vi "roi_selection multi.vi"(7 "Peak selected":i32, 8 "List Parameter Fit In":dbl[][](array[numeric]), 9 "List ROI In":dbl[][](array[numeric]), 10 "List Peaks":string[][](table), 11 "Spectrum In":cluster{"Locations":dbl[], "Amplitudes":dbl[]}) -> (2 "List Parameter Fit Out":dbl[][](array[numeric]), 3 "List ROI Out":dbl[][](array[numeric]))   [LabVIEW 2020]
uses:
  <vilib>/Analysis/NI_AALPro.lvlib
  <vilib>/Analysis/6fits.llb/Curve Fitting Criteria.ctl
panel:
  out "Parameters Fit":T1
  out "standard deviation":dbl
  out "FWHM":dbl
  out "amplitude":dbl
  out "XY Graph 2":cluster{dbl[], "Best Gaussian Fit":dbl[]}[](graph)
  in  "Elements":string[][](table)
  out "XY Graph":cluster{"Channels":dbl[], "Intensity":dbl[]}(graph)
  out "Spectrum":cluster{"Locations":dbl[], "Amplitudes":dbl[]}(graph)
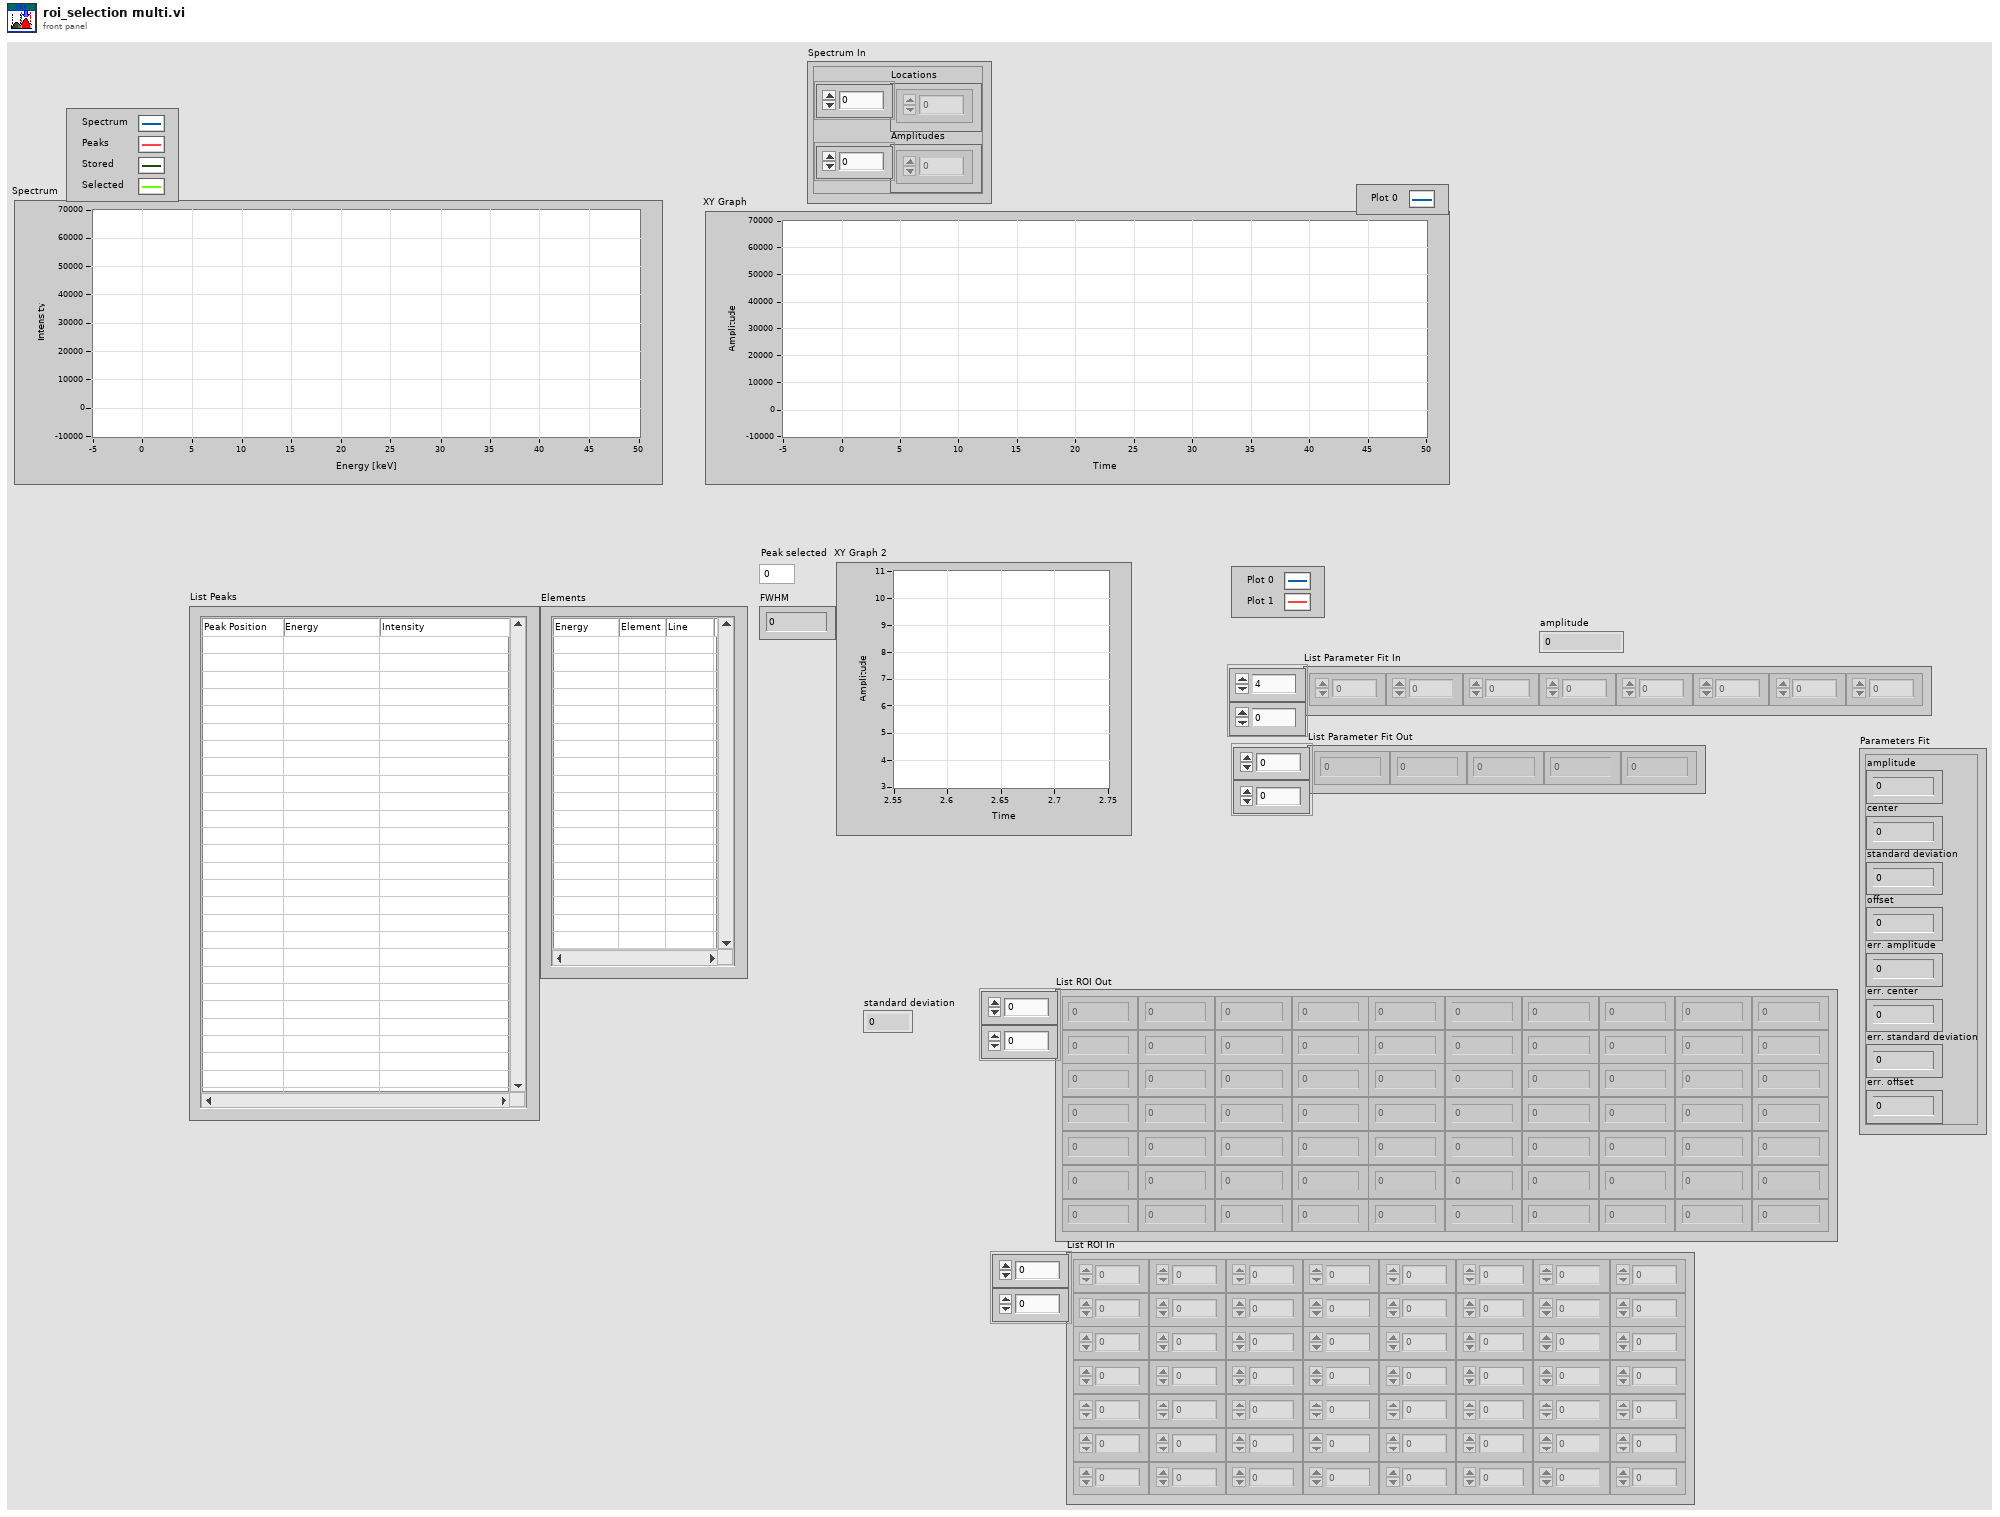
[diagram p1: front panel]
types:
  T1 = cluster{"amplitude":dbl, "center":dbl, "standard deviation":dbl, "offset":dbl, "err. amplitude":dbl, "err. center":dbl, "err. standard deviation":dbl, "err. offset":dbl}
  T2 = cluster{"initial amplitude":dbl, "initial center":dbl, "initial standard deviation":dbl, "offset":dbl}
  T3 = typedef "NI_AALPro.lvlib/Curve Fitting Criteria.ctl" = u16
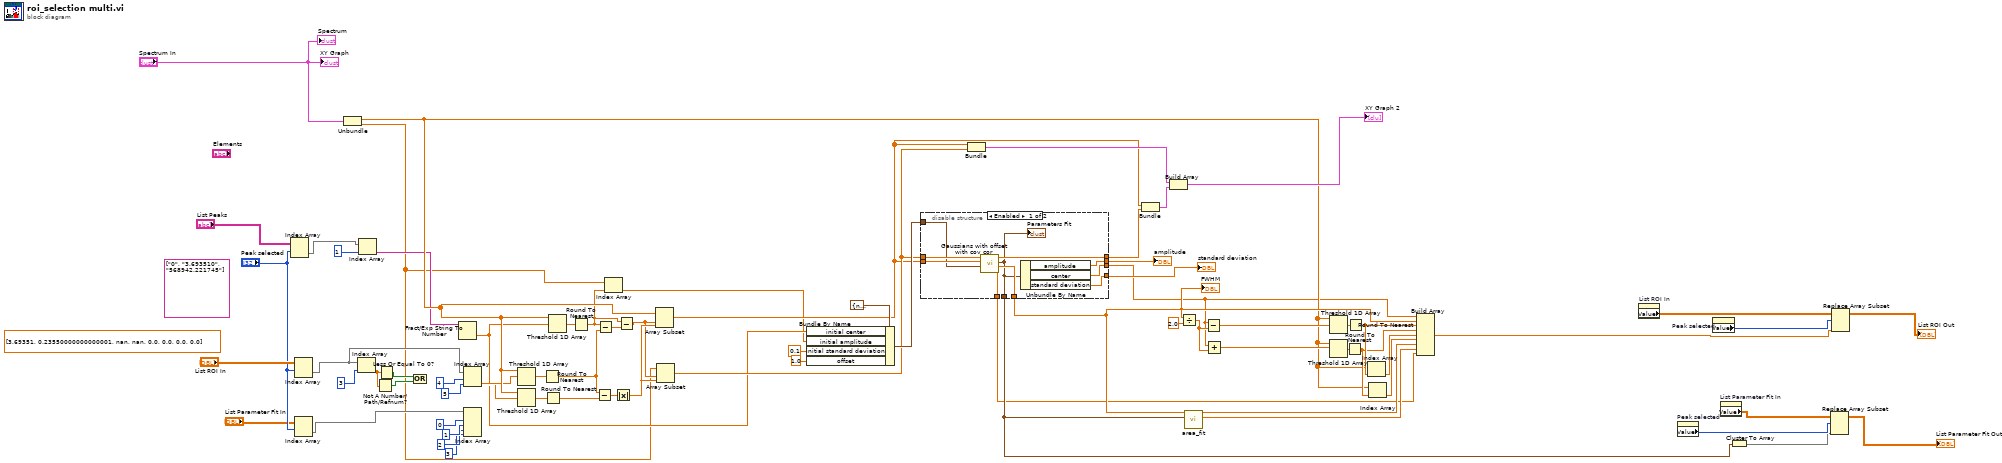
[diagram p0: block diagram]
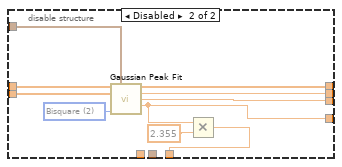
[diagram p2: hidden frame]
diagram:
  (unwired) dbl[][] [[3.69351, 0.23550000000000001, nan, nan, 0.0, 0.0, 0.0, 0.0]] ("List ROI In")
  (unwired) string[][] [["0", "3.693510", "568942.221745"]] ("List Peaks 2")
  n1 = Index Array(array="List Peaks", index (row)="Peak selected") -> (element=w70:string[])  [unwired: 1 in]
  n2 = Index Array(array="List Parameter Fit In", index (row)="Peak selected") -> (element=w65:dbl[])  [unwired: 1 in]
  n3 = Index Array(array="List ROI In", index (row)="Peak selected") -> (element=w68:dbl[])  [unwired: 1 in]
  n4 = Unbundle("Spectrum In") -> ("Locations"=w40:dbl[], "Amplitudes"=w5:dbl[])
  n5 = Index Array(array=w68, index=3) -> (element=w42:dbl)
  n6 = Index Array(array=w70, index=1 ("disabled index (col)")) -> (element=w7:string)
  n7 = Not A Number/Path/Refnum?(number/path/refnum=w42) -> (NaN/Path/Refnum?=w41:bool)
  n8 = Less Or Equal To 0?(x=w42) -> (x <= 0?=w43:bool)
  n9 = Compound Arithmetic op=OR(w43, w41) -> ()  [unwired: 1 out]
  n10 = Fract/Exp String To Number(string=w7) -> (number=w6:dbl)  [unwired: 3 in, 1 out]
  n11 = Index Array(array=w68, index #1=4 ("disabled index (col)"), index #2=5 ("disabled index (col)")) -> (element #1=w30:dbl, element #2=w27:dbl)
  n12 = Index Array(array=w65, index #1=0 ("index (col)"), index #2=1 ("index (col)"), index #3=2 ("index (col)"), index #4=3 ("index (col)")) -> ()  [unwired: 4 out]
  n13 = Threshold 1D Array(2:w30, 3:w40) -> (0:w28:dbl)  [unwired: 1 in]
  n14 = Threshold 1D Array(2:w27, 3:w40) -> (0:w29:dbl)  [unwired: 1 in]
  n15 = Round To Nearest(number=w28) -> (nearest integer value=w25:dbl)
  n16 = Round To Nearest(number=w29) -> (nearest integer value=w26:dbl)
  n17 = Threshold 1D Array(2:w6, 3:w40) -> (0:w33:dbl)  [unwired: 1 in]
  n18 = Round To Nearest(number=w33) -> (nearest integer value=w4:dbl)
  n19 = Subtract(x=w25, y=w26) -> (x-y=w32:dbl)
  n20 = Subtract(x=w4, y=w25) -> (x-y=w24:dbl)
  n21 = Index Array(array=w5, index=w4) -> (element=w3:dbl)
  n22 = Absolute Value(x=w32) -> (abs(x)=w31:dbl)
  n23 = Subtract(x=w4, y=w24) -> (x-y=w23:dbl)
  n24 = Array Subset(array=w40, index=w23, length=w31) -> (w36:dbl[])
  n25 = Array Subset(array=w5, index=w23, length=w31) -> (w37:dbl[])
  n26 = Bundle By Name(cluster=T2 {"initial amplitude"=nan, "initial center"=nan, "initial standard deviation"=nan, "offset"=nan} ("initial guess"), "initial center"=w6, "initial amplitude"=w3, "initial standard deviation"=0.1, "offset"=1.0) -> (w38:T2)
  n27 = disable-structure shown="Enabled" {
    disable-tunnel: w38 -> [w80 w92]
    disable-tunnel: [w79 w91] -> w64
    disable-tunnel: w36 -> [w81 w90]
    disable-tunnel: w37 -> [w82 w89]
    disable-tunnel: [w74 w84] -> w49
    disable-tunnel: [w75 w87] -> w35
    disable-tunnel: [w76 w86] -> w48
    disable-tunnel: [w78 w83] -> w46
    disable-tunnel: [w77 _] -> w44
    disable-tunnel: [w73 _] -> w34
    frame Enabled {
      n28 = call "Gaussians with offset with cov cor.vi"("initial guess"=w80, "X"=w81, "Y"=w82) -> ("R-square"=w73:dbl, "FWHM"=w78:dbl, "Parameters Fit"=w77:T1, "best nonlinear fit"=w79:dbl[])  [unwired: 5 in]
      "Parameters Fit" <- w77
      n29 = Unbundle By Name(w77) -> ("amplitude"=w76:dbl, "center"=w75:dbl, "standard deviation"=w74:dbl)
    }
    frame Disabled {
      w88 = T3 2 items=["Least Square", "Least Absolute Residual", "Bisquare"] ("method")
      n30 = call <vilib>:"Gaussian Peak Fit.vi"("Y"=w89, "initial guess"=w92, "X"=w90, "method"=w88) -> ("Best Gaussian Fit"=w91:dbl[], "amplitude"=w86:dbl, "center"=w87:dbl, "standard deviation"=w84:dbl)  [unwired: 5 in, 3 out]
      n31 = Multiply(x=w84, y=2.355) -> (x*y=w83:dbl)
    }
  }
  "amplitude" <- w48
  "FWHM" <- w46
  "standard deviation" <- w49
  n32 = Bundle(w36, w37) -> (w62:cluster{dbl[], dbl[]})  [unwired: 1 in]
  n33 = Bundle(w36, "best nonlinear fit"=w64) -> (w63:cluster{dbl[], "best nonlinear fit":dbl[]})  [unwired: 1 in]
  n34 = Build Array(w62, w63) -> (→"XY Graph 2":cluster{dbl[], "best nonlinear fit":dbl[]}[])
  n35 = Divide(x=w46, y=2.0) -> (x/y=w60:dbl)
  n36 = call "area_fit.vi"("Parameters Fit"=w44, "FWHM"=w46) -> ("Err. Area"=w45:dbl, "Area"=w47:dbl)  [unwired: 8 in]
  n37 = Subtract(x=w35, y=w60) -> (x-y=w58:dbl)
  n38 = Add(x=w35, y=w60) -> (x+y=w59:dbl)
  n39 = Threshold 1D Array(2:w58, 3:w40) -> (0:w57:dbl)  [unwired: 1 in]
  n40 = Threshold 1D Array(2:w59, 3:w40) -> (0:w56:dbl)  [unwired: 1 in]
  n41 = Round To Nearest(number=w56) -> (nearest integer value=w52:dbl)
  n42 = Round To Nearest(number=w57) -> (nearest integer value=w53:dbl)
  n43 = Index Array(array=w40, index=w53) -> (element=w51:dbl)
  n44 = Index Array(array=w40, index=w52) -> (element=w50:dbl)
  n45 = Build Array(w35, w46, w53, w52, w51, w50, w47, w45, w34) -> (w13:dbl[])
  n46 = property on="List ROI In" class="Arr (strict)"() -> ("Value"=w15:dbl[][])  [unwired: 2 in, 2 out]
  n47 = property on="Peak selected" class="DigNum (strict)"() -> ("Value"=w10:i32)  [unwired: 2 in, 2 out]
  n48 = property on="Peak selected" class="DigNum (strict)"() -> ("Value"=w14:i32)  [unwired: 2 in, 2 out]
  n49 = property on="List Parameter Fit In" class="Arr (strict)"() -> ("Value"=w11:dbl[][])  [unwired: 2 in, 2 out]
  n50 = Cluster To Array(cluster=w44) -> (array=w9:dbl[])
  n51 = Replace Array Subset(array=w11, new element=w9, index (row)=w10) -> (→"List Parameter Fit Out":dbl[][])  [unwired: 1 in]
  n52 = Replace Array Subset(array=w15, new element=w13, index (row)=w14) -> (→"List ROI Out":dbl[][])  [unwired: 1 in]
  "Spectrum" <- "Spectrum In"
  "XY Graph" <- "Spectrum In"
